vi "solar_visa VISA Timeout.vi"(8 "error in (no error)":errorcluster, 10 "VISA Timeout (0 = Ignore)":u32, 11 "VISA Resource in":refnum<visa-resource-name>) -> (0 "error out":errorcluster, 2 "old VISA Timeout":u32, 3 "VISA Resource out":refnum<visa-resource-name>)   [LabVIEW 2018]
doc: "This sets the VISA timeout and returns the previous timeout value."
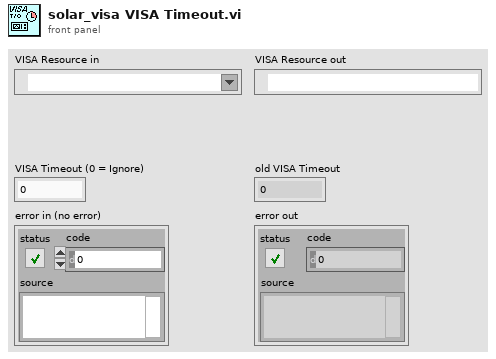
[diagram p1: front panel]
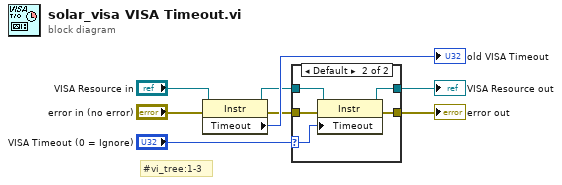
[diagram p0: block diagram]
diagram:
  # "#vi_tree:1-3"
  n1 = property class="Instr"(reference="VISA Resource in", error in="error in (no error)") -> (reference out=w1:refnum<visa-resource-name>, error out=w2:errorcluster, "Timeout"=→"old VISA Timeout":u32)
  n2 = case shown="Default" "VISA Timeout (0 = Ignore)" {
    selector: "VISA Timeout (0 = Ignore)" -> [_ w11]
    tunnel: w2 -> [w9 w15]
    tunnel: [w9 w14] -> w6
    tunnel: w1 -> [w10 w13]
    tunnel: [w10 w12] -> w5
    frame 0 {
    }
    frame Default {
      n3 = property class="Instr"(reference=w13, error in=w15, "Timeout"=w11) -> (reference out=w12:refnum<visa-resource-name>, error out=w14:errorcluster)
    }
  }
  "error out" <- w6
  "VISA Resource out" <- w5
